vi "VPA QC XDCR Setup.vi"(9 "DAQ Ref Cluster":T1) -> ()   [LabVIEW 2013]
uses:
  Controls/VPA QC DAQ Ref Cluster.ctl
panel:
  in  "Cancel":bool
  in  "OK":bool
  out "XDCR 2 PSI":dbl
  out "XDCR 2 Volts":dbl
  out "XDCR 1 PSI":dbl
  out "XDCR 1 Volts":dbl
  in  "Transducer 2\nScale Factor":dbl
  in  "Transducer 1 \nScale Factor":dbl
  in  "Transducer 2\nOffset":dbl
  in  "Transducer 1\n Offset":dbl
  # "Transducer Calibration"
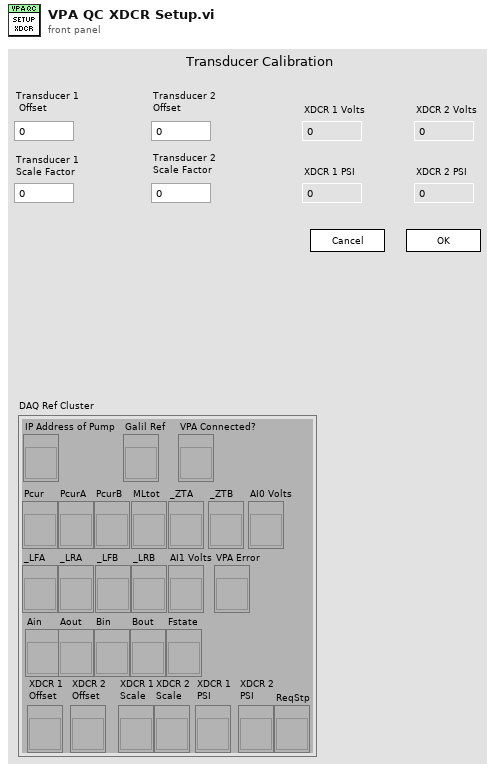
[diagram p1: front panel]
types:
  T1 = typedef "VPA QC DAQ Ref Cluster.ctl" = cluster{"IP Address of Pump":refnum<vi>, "Galil Ref":refnum<vi>, "VPA Connected?":refnum<vi>, "Pcur":refnum<vi>, "PcurA":refnum<vi>, "PcurB":refnum<vi>, "MLtot":refnum<vi>, "_LFA":refnum<vi>, "_LRA":refnum<vi>, "_LFB":refnum<vi>, "_LRB":refnum<vi>, "_ZTA":refnum<vi>, "_ZTB":refnum<vi>, "AI0 Volts":refnum<vi>, "AI1 Volts":refnum<vi>, "VPA Error":refnum<vi>, "Ain":refnum<vi>, "Aout":refnum<vi>, "Bin":refnum<vi>, "Bout":refnum<vi>, "Fstate":refnum<vi>, "XDCR 1\nOffset":refnum<vi>, "XDCR 2 \nOffset":refnum<vi>, "XDCR 1\nScale":refnum<vi>, "XDCR 2\nScale":refnum<vi>, "XDCR 1\nPSI":refnum<vi>, "XDCR 2\nPSI":refnum<vi>, "ReqStp":refnum<vi>}
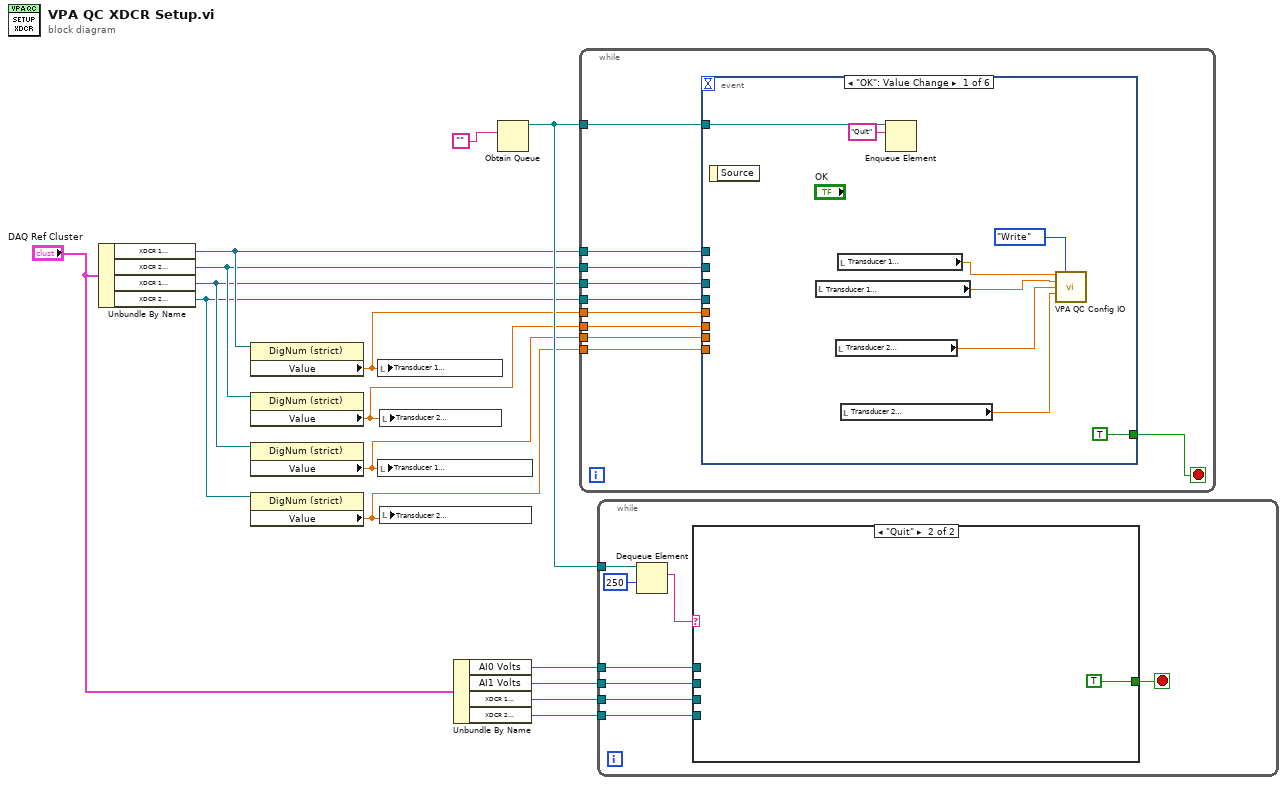
[diagram p0: block diagram]
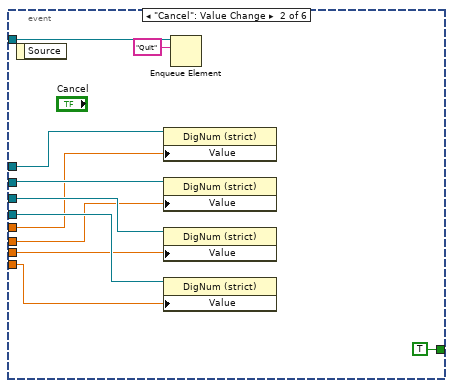
[diagram p2: hidden frame]
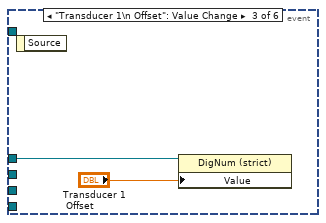
[diagram p3: hidden frame]
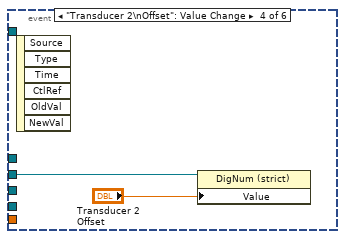
[diagram p4: hidden frame]
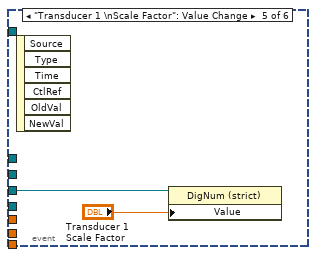
[diagram p5: hidden frame]
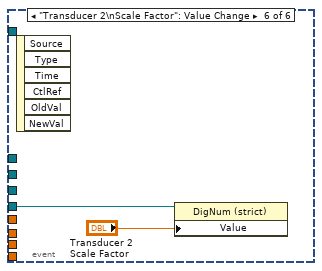
[diagram p6: hidden frame]
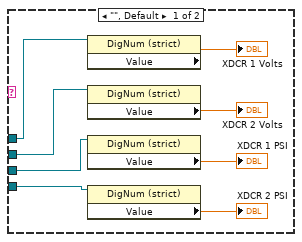
[diagram p7: hidden frame]
diagram:
  n1 = Unbundle By Name("DAQ Ref Cluster") -> ("XDCR 1\nOffset"=w8:refnum<vi>, "XDCR 2 \nOffset"=w7:refnum<vi>, "XDCR 1\nScale"=w6:refnum<vi>, "XDCR 2\nScale"=w5:refnum<vi>)
  n2 = property class="DigNum (strict)"(reference=w8) -> ("Value"=w4:dbl)  [unwired: 1 in, 2 out]
  n3 = property class="DigNum (strict)"(reference=w7) -> ("Value"=w3:dbl)  [unwired: 1 in, 2 out]
  n4 = property class="DigNum (strict)"(reference=w6) -> ("Value"=w2:dbl)  [unwired: 1 in, 2 out]
  n5 = property class="DigNum (strict)"(reference=w5) -> ("Value"=w1:dbl)  [unwired: 1 in, 2 out]
  n6 = local write "Transducer 1\n Offset"(w4) -> ()
  n7 = local write "Transducer 1 \nScale Factor"(w2) -> ()
  n8 = local write "Transducer 2\nOffset"(w3) -> ()
  n9 = local write "Transducer 2\nScale Factor"(w1) -> ()
  n10 = Unbundle By Name("DAQ Ref Cluster") -> ("AI0 Volts"=w13:refnum<vi>, "AI1 Volts"=w12:refnum<vi>, "XDCR 1\nPSI"=w11:refnum<vi>, "XDCR 2\nPSI"=w10:refnum<vi>)
  n11 = Obtain Queue(element data type="") -> (queue out=w14:refnum<queue>)  [unwired: 4 in, 2 out]
  n12 = while {
    tunnel: w14 -> [w20]
    tunnel: w8 -> [w24]
    tunnel: w7 -> [w23]
    tunnel: w6 -> [w22]
    tunnel: w5 -> [w21]
    tunnel: w4 -> [w19]
    tunnel: w3 -> [w18]
    tunnel: w2 -> [w16]
    tunnel: w1 -> [w17]
    stop <- w25 stop-if-true
    n13 = event shown="[0] \"OK\": Value Change" {
      selector: _ -> [_ _ _ _ _ _]
      dyn-events: _ -> [_ _ _ _ _ _]
      timeout: _ -> [_ _ _ _ _ _]
      tunnel: [TRUE TRUE _ _ _ _] -> w25
      tunnel: w24 -> [_ w42 w46 _ _ _]
      tunnel: w23 -> [_ w41 _ w48 _ _]
      tunnel: w22 -> [_ w40 _ _ w50 _]
      tunnel: w21 -> [_ w39 _ _ _ w52]
      tunnel: w20 -> [w32 w44 _ _ _ _]
      tunnel: w19 -> [_ w38 _ _ _ _]
      tunnel: w18 -> [_ w37 _ _ _ _]
      tunnel: w17 -> [_ w35 _ _ _ _]
      tunnel: w16 -> [_ w36 _ _ _ _]
      event "OK": Value Change {
        n14 = event-data() -> ()  [unwired: 1 in, 1 out]
        n15 = local read "Transducer 1 \nScale Factor"() -> (w28:dbl)
        n16 = local read "Transducer 2\nOffset"() -> (w27:dbl)
        n17 = local read "Transducer 1\n Offset"() -> (w29:dbl)
        n18 = local read "Transducer 2\nScale Factor"() -> (w26:dbl)
        n19 = Enqueue Element(queue=w32, element="Quit") -> ()  [unwired: 2 in, 3 out]
        n20 = call "VPA QC Config IO.vi"("XDCR 1 Offset"=w29, "Function"=enum16{"Read", "Write"}."Write", "XDCR 1 Scale"=w28, "XDCR 2 Offset"=w27, "XDCR 2 Scale"=w26) -> ()  [unwired: 7 in, 4 out]
      }
      event "Cancel": Value Change {
        n21 = event-data() -> ()  [unwired: 1 in, 1 out]
        n22 = property class="DigNum (strict)"(reference=w42, "Value"=w38) -> ()  [unwired: 1 in, 2 out]
        n23 = property class="DigNum (strict)"(reference=w41, "Value"=w37) -> ()  [unwired: 1 in, 2 out]
        n24 = property class="DigNum (strict)"(reference=w40, "Value"=w36) -> ()  [unwired: 1 in, 2 out]
        n25 = property class="DigNum (strict)"(reference=w39, "Value"=w35) -> ()  [unwired: 1 in, 2 out]
        n26 = Enqueue Element(queue=w44, element="Quit") -> ()  [unwired: 2 in, 3 out]
      }
      event "Transducer 1\n Offset": Value Change {
        n27 = event-data() -> ()  [unwired: 1 in, 1 out]
        n28 = property class="DigNum (strict)"(reference=w46, "Value"="Transducer 1\n Offset") -> ()  [unwired: 1 in, 2 out]
      }
      event "Transducer 2\nOffset": Value Change {
        n29 = event-data() -> ()  [unwired: 1 in, 6 out]
        n30 = property class="DigNum (strict)"(reference=w48, "Value"="Transducer 2\nOffset") -> ()  [unwired: 1 in, 2 out]
      }
      event "Transducer 1 \nScale Factor": Value Change {
        n31 = event-data() -> ()  [unwired: 1 in, 6 out]
        n32 = property class="DigNum (strict)"(reference=w50, "Value"="Transducer 1 \nScale Factor") -> ()  [unwired: 1 in, 2 out]
      }
      event "Transducer 2\nScale Factor": Value Change {
        n33 = event-data() -> ()  [unwired: 1 in, 6 out]
        n34 = property class="DigNum (strict)"(reference=w52, "Value"="Transducer 2\nScale Factor") -> ()  [unwired: 1 in, 2 out]
      }
    }
  }
  n35 = while {
    tunnel: w14 -> [w60]
    tunnel: w13 -> [w55]
    tunnel: w12 -> [w54]
    tunnel: w11 -> [w56]
    tunnel: w10 -> [w53]
    stop <- w57 stop-if-true
    n36 = Dequeue Element(queue=w60, timeout in ms (-1)=250) -> (element=w59:string)  [unwired: 1 in, 3 out]
    n37 = case shown="\"Quit\"" w59 {
      tunnel: [_ TRUE] -> w57
      tunnel: w56 -> [w66 _]
      tunnel: w55 -> [w68 _]
      tunnel: w54 -> [w67 _]
      tunnel: w53 -> [w65 _]
      frame "", Default {
        n38 = property class="DigNum (strict)"(reference=w68) -> ("Value"=→"XDCR 1 Volts":dbl)  [unwired: 1 in, 2 out]
        n39 = property class="DigNum (strict)"(reference=w67) -> ("Value"=→"XDCR 2 Volts":dbl)  [unwired: 1 in, 2 out]
        n40 = property class="DigNum (strict)"(reference=w66) -> ("Value"=→"XDCR 1 PSI":dbl)  [unwired: 1 in, 2 out]
        n41 = property class="DigNum (strict)"(reference=w65) -> ("Value"=→"XDCR 2 PSI":dbl)  [unwired: 1 in, 2 out]
      }
      frame "Quit" {
      }
    }
  }
